vi "Rubix Number Array to Text Array.vi"(11 "Cube Orientation":string[][](array[string])) -> (3 "Text Array":string[][](array[string])=[["o0", "r0", "y0", "r1", "r2", "g0", "r3", "w0", "w1"], ["o1", "y1", "b0", "w2", "y2", "r4", "b1", "o2", "o3"], ["o4", "y3", "r5", "g1", "o5", "o6", "w3", "o7", "r6"], ["g2", "w4", "g3", "g4", "w5", "w6", "g5", "y4", "y5"], ["y6", "b2", "w7", "b3", "b4", "g6", "y7", "b5", "b6"], ["b7", "o8", "r7", "r8", "g7", "y8", "w8", "b8", "g8"]])   [LabVIEW 2019]
panel:
  # "White=0\nRed=1\nOrange=2\nYello=3\nGreen=4\nBlue=5"
  # "F\nR\nB\nL\nU\nD"
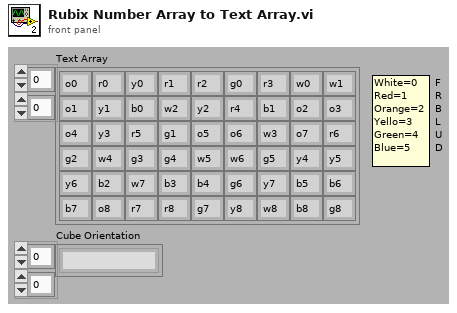
[diagram p1: front panel]
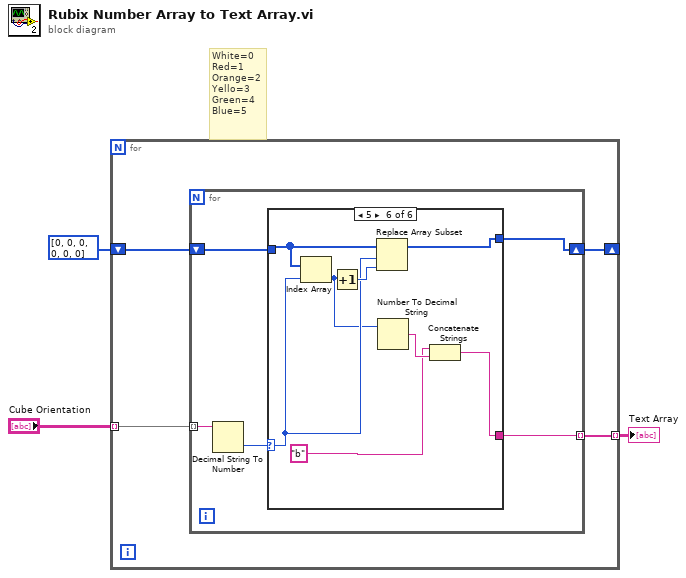
[diagram p0: block diagram]
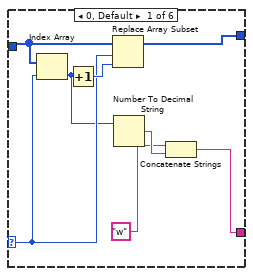
[diagram p2: hidden frame]
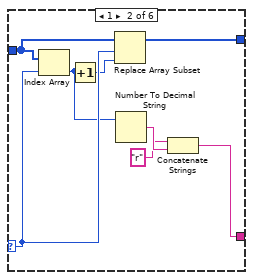
[diagram p3: hidden frame]
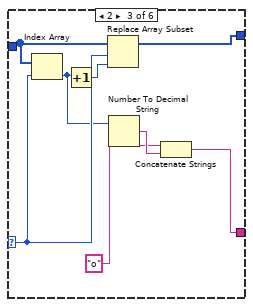
[diagram p4: hidden frame]
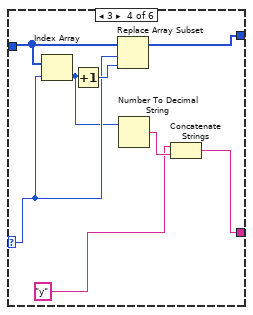
[diagram p5: hidden frame]
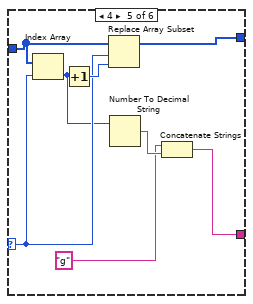
[diagram p6: hidden frame]
diagram:
  # "White=0\nRed=1\nOrange=2\nYello=3\nGreen=4\nBlue=5"
  n1 = for {
    tunnel: "Cube Orientation" -> [w7] mode=indexing
    shift-right: [w5] -> _
    shift-left: i32[] [0, 0, 0, 0, 0, 0] -> [w6]
    tunnel: [w4] -> w2 mode=indexing
    n2 = for {
      tunnel: w7 -> [w9] mode=indexing
      shift-right: [w11] -> w5
      shift-left: w6 -> [w12]
      tunnel: [w10] -> w4 mode=indexing
      n3 = Decimal String To Number(string=w9) -> (number=w8:i32)  [unwired: 2 in, 1 out]
      n4 = case shown="5" w8 {
        selector: w8 -> [w16 w28 w32 w41 w49 w54]
        tunnel: [w14 w22 w30 w38 w46 w56] -> w10
        tunnel: w12 -> [w17 w27 w31 w40 w48 w55]
        tunnel: [w18 w26 w34 w42 w50 w58] -> w11
        frame 0, Default {
          n5 = Index Array(array=w17, index=w16) -> (element=w13:i32)
          n6 = Increment(x=w13) -> (x+1=w19:i32)
          n7 = Replace Array Subset(array=w17, new element=w19, index=w16) -> (w18:i32[])
          n8 = Number To Decimal String(number=w13) -> (decimal integer string=w20:string)  [unwired: 1 in]
          n9 = Concatenate Strings("w", w20) -> (w14:string)
        }
        frame 1 {
          n10 = Index Array(array=w27, index=w28) -> (element=w21:i32)
          n11 = Increment(x=w21) -> (x+1=w25:i32)
          n12 = Replace Array Subset(array=w27, new element=w25, index=w28) -> (w26:i32[])
          n13 = Number To Decimal String(number=w21) -> (decimal integer string=w24:string)  [unwired: 1 in]
          n14 = Concatenate Strings("r", w24) -> (w22:string)
        }
        frame 2 {
          n15 = Index Array(array=w31, index=w32) -> (element=w29:i32)
          n16 = Increment(x=w29) -> (x+1=w35:i32)
          n17 = Replace Array Subset(array=w31, new element=w35, index=w32) -> (w34:i32[])
          n18 = Number To Decimal String(number=w29) -> (decimal integer string=w36:string)  [unwired: 1 in]
          n19 = Concatenate Strings("o", w36) -> (w30:string)
        }
        frame 3 {
          n20 = Index Array(array=w40, index=w41) -> (element=w37:i32)
          n21 = Increment(x=w37) -> (x+1=w43:i32)
          n22 = Replace Array Subset(array=w40, new element=w43, index=w41) -> (w42:i32[])
          n23 = Number To Decimal String(number=w37) -> (decimal integer string=w44:string)  [unwired: 1 in]
          n24 = Concatenate Strings("y", w44) -> (w38:string)
        }
        frame 4 {
          n25 = Index Array(array=w48, index=w49) -> (element=w45:i32)
          n26 = Increment(x=w45) -> (x+1=w51:i32)
          n27 = Replace Array Subset(array=w48, new element=w51, index=w49) -> (w50:i32[])
          n28 = Number To Decimal String(number=w45) -> (decimal integer string=w52:string)  [unwired: 1 in]
          n29 = Concatenate Strings("g", w52) -> (w46:string)
        }
        frame 5 {
          n30 = Index Array(array=w55, index=w54) -> (element=w53:i32)
          n31 = Increment(x=w53) -> (x+1=w59:i32)
          n32 = Replace Array Subset(array=w55, new element=w59, index=w54) -> (w58:i32[])
          n33 = Number To Decimal String(number=w53) -> (decimal integer string=w60:string)  [unwired: 1 in]
          n34 = Concatenate Strings("b", w60) -> (w56:string)
        }
      }
    }
  }
  "Text Array" <- w2
